vi "Set AO Voltage.vi"(0 "RedPitaya connection in":refnum<k5>, 2 "Pin #":u16(ring) items=["AOUT0", "AOUT1", "AOUT2", "AOUT3"], 3 "Analog Voltage Value":dbl min=0.0 max=1.8, 5 "error in":errorcluster, 12 "timeout ms (2000)":i32=2000) -> (14 "RedPitaya connection out":refnum<k5>, 19 "error out":errorcluster)   [LabVIEW 2010, in "RedPitaya.lvlib"]
doc: "Set analog voltage on slow analog outputs. Voltage range of slow analog outputs is: 0-1.8V"
uses:
  RedPitaya.lvlib
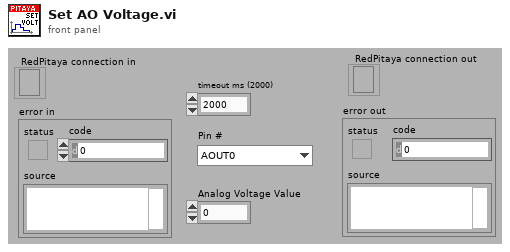
[diagram p1: front panel]
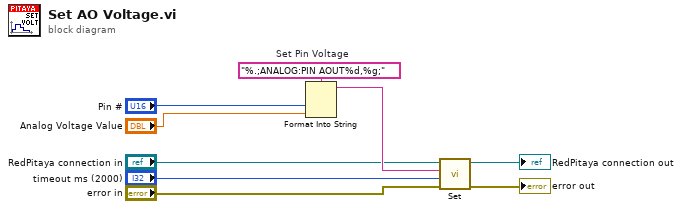
[diagram p0: block diagram]
diagram:
  w9 = "%.;ANALOG:PIN AOUT%d,%g;"  # Set Pin Voltage
  n1 = Format Into String(format string=w9, "Pin #", "Analog Voltage Value") -> (resulting string=w8:string)  [unwired: 2 in, 1 out]
  n2 = call "Set.vi"("error in"="error in", "timeout ms (2000)"="timeout ms (2000)", "SCPI Message"=w8, "RedPitaya connection in"="RedPitaya connection in") -> ("error out"=→"error out":errorcluster, "RedPitaya connection out"=→"RedPitaya connection out":refnum<k5>)  [unwired: 5 in, 1 out]
